vi "Solve Linear Equations (multiple right hand).vi"(2 "matrix type":T1, 3 "Known Matrix":T2, 4 "Input Matrix":T2) -> (0 "error":i32, 1 "Solution Matrix":T2)   [LabVIEW 2020, in "NI_AALPro.lvlib"]
doc: "Solves a linear system AX = Y. The data types you wire to the <B>Input Matrix</B> and <B>Known Vector</B> inputs determine the polymorphic instance to use."
uses:
  NI_AALPro.lvlib
  RealMatrix.ctl
  Matrix Type of Inverse Matrix.ctl
  <resource>/lvanlys.dll
  NI_Matrix.lvlib
  NI_AALBase.lvlib
panel:
  # "Solve Linear Equations"
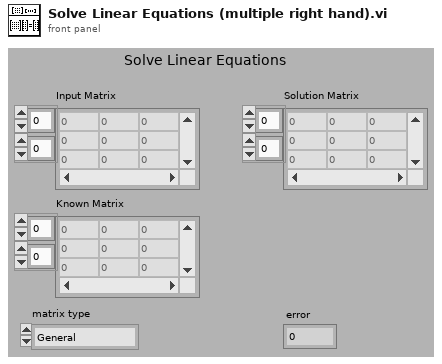
[diagram p1: front panel]
types:
  T1 = typedef "NI_AALBase.lvlib/Matrix Type of Inverse Matrix.ctl" = enum32{"General", "Positive Definite", "Lower Triangular", "Upper Triangular"}
  T2 = typedef "NI_Matrix.lvlib/RealMatrix.ctl" = dbl[][]
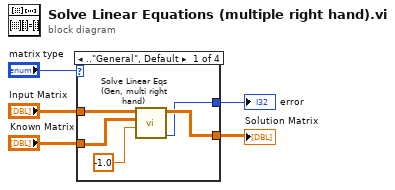
[diagram p0: block diagram]
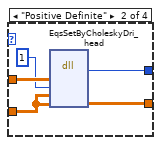
[diagram p2: hidden frame]
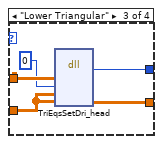
[diagram p3: hidden frame]
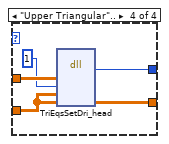
[diagram p4: hidden frame]
diagram:
  n1 = case shown="..\"General\", Default" "matrix type" {
    tunnel: "Known Matrix" -> [w9 w13 w19 w23]
    tunnel: "Input Matrix" -> [w10 w15 w20 w25]
    tunnel: [w7 w12 w18 w22] -> w2
    tunnel: [w6 w11 w17 w21] -> w1
    frame .."General", Default {
      n2 = call "Solve Linear Eqs (Gen, multi right hand).vi"("relative tolerance"=-1.0 ("relativeTol"), "Known Matrix"=w9, "Input Matrix"=w10) -> ("error"=w6:i32, "Solution Matrix"=w7:T2)  [unwired: 7 in]
    }
    frame "Positive Definite" {
      n3 = dll-call lib="C:/Program Files (x86)/National Instruments/LabVIEW 2020/resource/lvanlys.*" fn="EqsSetByCholeskyDri_head"("Input Matrix"=w15, "uplo"=1, "Known Matrix"=w13, "Known Matrix"=w13) -> (w11:i32, "Known Matrix"=w12:T2)  [unwired: 6 in, 2 out]
    }
    frame "Lower Triangular" {
      n4 = dll-call lib="C:/Program Files (x86)/National Instruments/LabVIEW 2020/resource/lvanlys.*" fn="TriEqsSetDri_head"("Input Matrix"=w20, "uplo"=0, "Known Matrix"=w19, "Known Matrix"=w19) -> (w17:i32, "Known Matrix"=w18:T2)  [unwired: 6 in, 2 out]
    }
    frame "Upper Triangular".. {
      n5 = dll-call lib="C:/Program Files (x86)/National Instruments/LabVIEW 2020/resource/lvanlys.*" fn="TriEqsSetDri_head"("Input Matrix"=w25, "uplo"=1, "Known Matrix"=w23, "Known Matrix"=w23) -> (w21:i32, "Known Matrix"=w22:T2)  [unwired: 6 in, 2 out]
    }
  }
  "error" <- w1
  "Solution Matrix" <- w2
